vi "FindWedgePrams.vi"(5 "P":T5={"x (cm)"=1.0, "y (cm)"=-3.0, "z (cm)"=1.0} {"x (cm)" format="%.2f"; "z (cm)" format="%.2f"; "y (cm)" format="%.2f"}, 7 "strip":T4={"radius (cm)"=10.0, "h (cm)"=2.0, "a (cm)"=6.0} {"radius (cm)" format="%.2f"; "a (cm)" format="%.2f"; "h (cm)" format="%.2f"}) -> (0 "variables":T1 {"Dtemp" format="%.2f"; "B" format="%.2f"; "A" format="%.2f"; "thetaw" format="%.2f"; "phih" format="%.2f"; "r (cm)" format="%.2f"}, 1 "Location Tests":T2, 2 "Case Number":i32, 3 "r values (cm)":T3 {"r5" format="%.2f"; "r4" format="%.4f"; "r3" format="%.4f"; "r2" format="%.4f"; "r1" format="%.2f"; "r0" format="%.2f"}, 4 "Transform matrix":dbl[][](array[numeric]) format="%.2f")   [LabVIEW 2022 SP3]
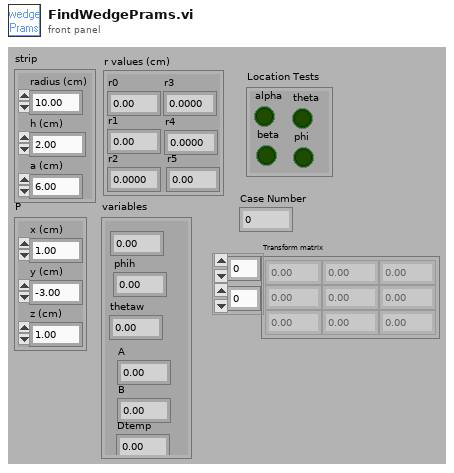
[diagram p1: front panel]
types:
  T1 = cluster{"r (cm)":dbl, "phih":dbl, "thetaw":dbl, "A":dbl, "B":dbl, "Dtemp":dbl}
  T2 = cluster{"alpha":bool, "beta":bool, "theta":bool, "phi":bool}
  T3 = cluster{"r0":dbl, "r1":dbl, "r2":dbl, "r3":dbl, "r4":dbl, "r5":dbl}
  T4 = cluster{"radius (cm)":dbl, "h (cm)":dbl, "a (cm)":dbl}
  T5 = cluster{"x (cm)":dbl, "y (cm)":dbl, "z (cm)":dbl}
  T6 = cluster{"r":dbl, "alphab":dbl, "thetab":dbl, "A":dbl, "B":dbl, "Dtemp":dbl}
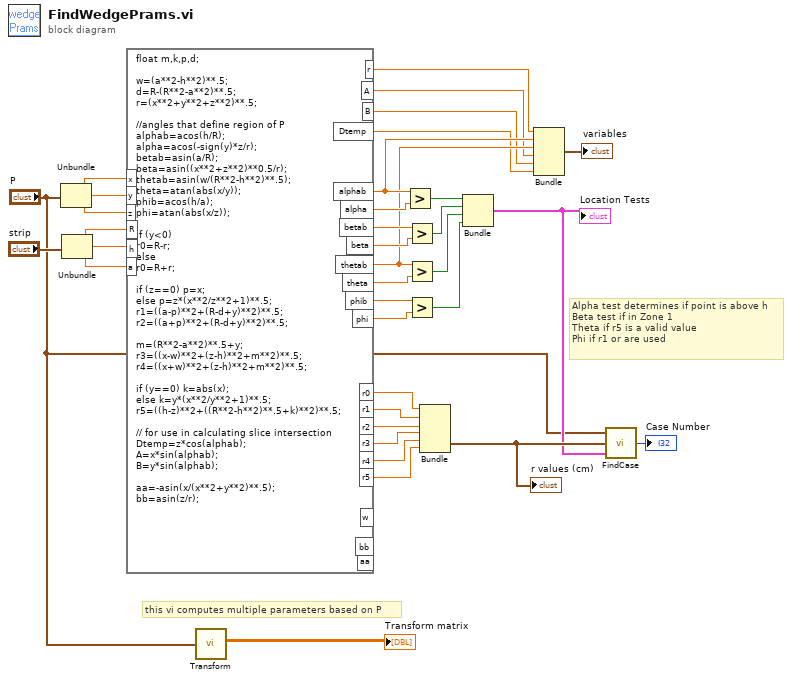
[diagram p0: block diagram]
diagram:
  # "Alpha test determines if point is above h\nBeta test if in Zone 1\nTheta if r5 is a valid value\nPhi if r1 or are used"
  # "this vi computes multiple parameters based on P"
  n1 = Unbundle("P") -> ("x (cm)"=w35:dbl, "y (cm)"=w34:dbl, "z (cm)"=w33:dbl)
  n2 = Unbundle("strip") -> ("radius (cm)"=w31:dbl, "h (cm)"=w30:dbl, "a (cm)"=w29:dbl)
  n3 = formula code="float m,k,p,d;\n\nw=(a**2-h**2)**.5;\nd=R-(R**2-a**2)**.5;\nr=(x**2+y**2+z**2)**.5;\n\n//angles that define region of P\nalphab=acos(h/R);\nalpha=acos(-sign(y)*z/r);\nbetab=asin(a/R);\nbeta=asin((x**2+z**2)**0.5/r);\nthetab=asin(w/(R**2-h**2)**.5);\ntheta=atan(abs(x/y));\nphib=acos(h/a);\nphi=atan(abs(x/z));\n\nif (y<0) \nr0=R-r;\nelse\nr0=R+r;\n\nif (z==0) p=x;\nelse p=z*(x**2/z**2+1)**.5;\nr1=((a-p)**2+(R-d+y)**2)**.5;\nr2=((a+p)**2+(R-d+y)**2)**.5;\n\nm=(R**2-a**2)**.5+y;\nr3=((x-w)**2+(z-h)**2+m**2)**.5;\nr4=((x+w)**2+(z-h)**2+m**2)**.5;\n\nif (y==0) k=abs(x);\nelse k=y*(x**2/y**2+1)**.5;\nr5=((h-z)**2+((R**2-h**2)**.5+k)**2)**.5;\n\n// for use in calculating slice intersection\nDtemp=z*cos(alphab);\nA=x*sin(alphab);\nB=y*sin(alphab);\n\naa=-asin(x/(x**2+y**2)**.5);\nbb=asin(z/r);"("z"=w33, "x"=w35, "y"=w34, "R"=w31, "a"=w29, "h"=w30) -> ("r0"=w26:dbl, "r1"=w27:dbl, "r2"=w28:dbl, "r3"=w25:dbl, "r4"=w24:dbl, "r5"=w23:dbl, "r"=w16:dbl, "alphab"=w15:dbl, "alpha"=w22:dbl, "beta"=w20:dbl, "betab"=w21:dbl, "thetab"=w14:dbl, "theta"=w19:dbl, "phib"=w18:dbl, "phi"=w17:dbl, "A"=w9:dbl, "B"=w8:dbl, "Dtemp"=w7:dbl)  [unwired: 3 out]
  n4 = call "Transform.vi"("P"="P") -> ("transfrom matrix"=→"Transform matrix":dbl[][])  [unwired: 4 out]
  n5 = Greater?(x=w15, y=w22) -> (0:w13:bool)
  n6 = Greater?(x=w21, y=w20) -> (0:w12:bool)
  n7 = Greater?(x=w14, y=w19) -> (0:w11:bool)
  n8 = Greater?(x=w18, y=w17) -> (0:w10:bool)
  n9 = Bundle("r0"=w26, "r1"=w27, "r2"=w28, "r3"=w25, "r4"=w24, "r5"=w23) -> (w6:T3)  [unwired: 1 out]
  "r values (cm)" <- w6
  n10 = Bundle(w13, w12, w11, w10) -> (w5:cluster{bool, bool, bool, bool})  [unwired: 1 out]
  "Location Tests" <- w5
  n11 = Bundle("r"=w16, "alphab"=w15, "thetab"=w14, "A"=w9, "B"=w8, "Dtemp"=w7) -> (→"variables":T6)  [unwired: 1 out]
  n12 = call "FindCase.vi"("Location Tests"=w5, "r values"=w6, "P"="P") -> ("Case Number"=→"Case Number":i32)
